vi "solar Delete COSMOS Files.vi"(8 "error in (no error)":errorcluster, 9 "Delete entire target folder? (F)":bool, 10 "Target Folders to Delete":string[](array[string]), 11 "COSMOS_Root":path) -> (0 "error out":errorcluster)   [LabVIEW 2018]
doc: "Deletes the COSMOS confiig targets files for cmdtlm.\n\nIf Delete entire target folder? is true, it will delete everything within the target folders. If it is false, it will just delete the cmd_tlm_server, and default cmd and tlm files."
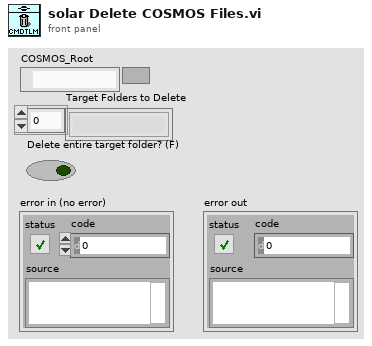
[diagram p1: front panel]
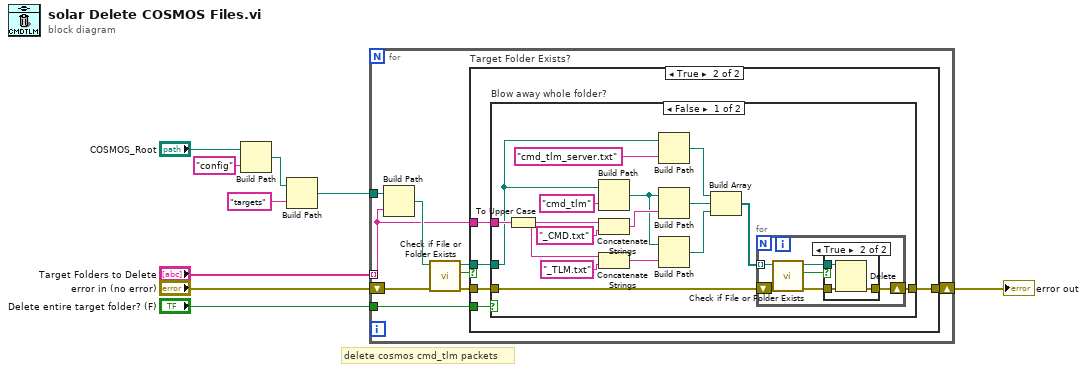
[diagram p0: block diagram]
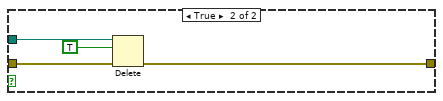
[diagram p4: hidden frame]
diagram:
  # "delete cosmos cmd_tlm packets"
  n1 = Build Path(base path="COSMOS_Root", name or relative path="config") -> (appended path=w3:path)
  n2 = Build Path(base path=w3, name or relative path="targets") -> (appended path=w6:path)
  n3 = for {
    shift-right: [w18] -> w8
    shift-left: "error in (no error)" -> [w14]
    tunnel: w6 -> [w17]
    tunnel: "Target Folders to Delete" -> [w10] mode=indexing
    tunnel: "Delete entire target folder? (F)" -> [w11]
    n4 = Build Path(base path=w17, name or relative path=w10) -> (appended path=w15:path)
    n5 = call <vilib>:"Check if File or Folder Exists.vi"("error in (no error)"=w14, "path"=w15) -> ("error out"=w13:errorcluster, "file or folder exists?"=w12:bool, "dup path"=w16:path)  [unwired: 7 in]
    n6 = case "Target Folder Exists?" shown="True" w12 {
      tunnel: [w19 w24] -> w18
      tunnel: w16 -> [_ w23]
      tunnel: w13 -> [w19 w22]
      tunnel: w11 -> [_ w21]
      tunnel: w10 -> [_ w20]
      frame False {
      }
      frame True {
        n7 = case "Blow away whole folder?" shown="False" w21 {
          tunnel: [w27 w53] -> w24
          tunnel: w23 -> [w31 w52]
          tunnel: w22 -> [w26 w51]
          tunnel: w20 -> [w38 _]
          frame False {
            n8 = To Upper Case(1:w38) -> (0:w35:string)
            n9 = Build Path(base path=w31, name or relative path="cmd_tlm") -> (appended path=w34:path)
            n10 = Concatenate Strings(w35, "_CMD.txt" ("string")) -> (w39:string)
            n11 = Concatenate Strings(w35, "_TLM.txt" ("string")) -> (w33:string)
            n12 = Build Path(base path=w31, name or relative path="cmd_tlm_server.txt") -> (appended path=w30:path)
            n13 = Build Path(base path=w34, name or relative path=w39) -> (appended path=w29:path)
            n14 = Build Path(base path=w34, name or relative path=w33) -> (appended path=w28:path)
            n15 = Build Array(w30, w29, w28) -> (w25:path[])
            n16 = for {
              shift-right: [w45] -> w27
              shift-left: w26 -> [w44]
              tunnel: w25 -> [w43] mode=indexing
              n17 = call <vilib>:"Check if File or Folder Exists.vi"("error in (no error)"=w44, "path"=w43) -> ("error out"=w46:errorcluster, "file or folder exists?"=w41:bool, "dup path"=w42:path)  [unwired: 7 in]
              n18 = case shown="True" w41 {
                tunnel: w46 -> [w47 w50]
                tunnel: [w47 w49] -> w45
                tunnel: w42 -> [_ w48]
                frame False {
                }
                frame True {
                  n19 = Delete(path (use dialog)=w48, error in=w50) -> (error out=w49:errorcluster)  [unwired: 3 in, 2 out]
                }
              }
            }
          }
          frame True {
            n20 = Delete(path (use dialog)=w52, entire hierarchy (F)=TRUE, error in=w51) -> (error out=w53:errorcluster)  [unwired: 2 in, 2 out]
          }
        }
      }
    }
  }
  "error out" <- w8
